vi "new.vi"(8 "error in (no error)":errorcluster, 11 "data":dbl) -> (0 "error out":errorcluster, 3 "Iterator out":refnum<class "Iterator.lvclass">)   [LabVIEW 2021, in "Iterator.lvclass"]
uses:
  Iterator.lvclass
  DoublyNode/DoublyNode.lvclass
  IDoublyNode/IDoublyNode.lvclass
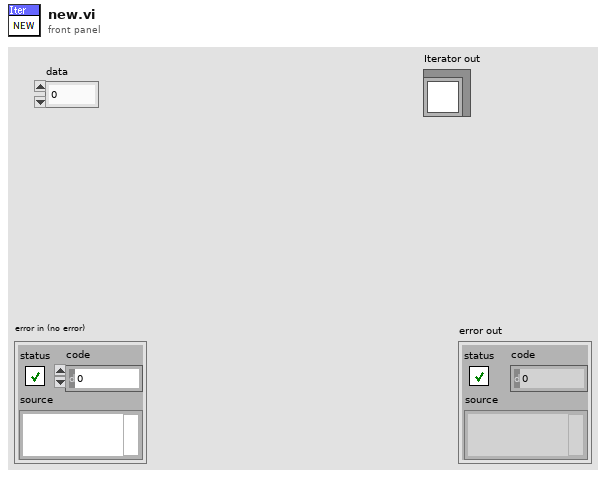
[diagram p1: front panel]
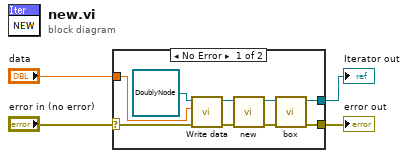
[diagram p0: block diagram]
diagram:
  n1 = case shown="No Error" "error in (no error)" {
    selector: "error in (no error)" -> [w12 w14]
    tunnel: [w6 w14] -> w3
    tunnel: "data" -> [w11 _]
    tunnel: [w5 _] -> w1
    frame No Error {
      n2 = call-dynamic "Write data.vi"("error in (no error)"=w12, "data"=w11, "DoublyNode in"=refnum<class "DoublyNode.lvclass"> refnum ("DoublyNode.lvclass")) -> ("error out"=w9:errorcluster, "DoublyNode out"=w10:refnum<class "DoublyNode.lvclass">)  [unwired: 7 in]
      n3 = call "new.vi"("error in (no error)"=w9, "IDoublyNode in"=w10) -> ("error out"=w7:errorcluster, "node ref"=w8:refnum<data-value>)  [unwired: 8 in]
      n4 = call "box.vi"("error in (no error)"=w7, "node"=w8) -> ("error out"=w6:errorcluster, "Iterator out"=w5:refnum<class "Iterator.lvclass">)  [unwired: 8 in]
    }
    frame Error {
    }
  }
  "error out" <- w3
  "Iterator out" <- w1
